vi "pidMotor.vi"(0 "Master refnum":string="My Motor RefNum", 5 "Slave refnum":string="My Motor RefNum", 7 "Joystick cluster":cluster{"X":dbl, "Y":dbl}, 9 "Speed Multiplier":dbl, 11 "error in (no error)":errorcluster) -> (4 "Set Velocity":dbl, 8 "Encoder Velocity":dbl, 15 "error out":errorcluster)   [LabVIEW 2014]
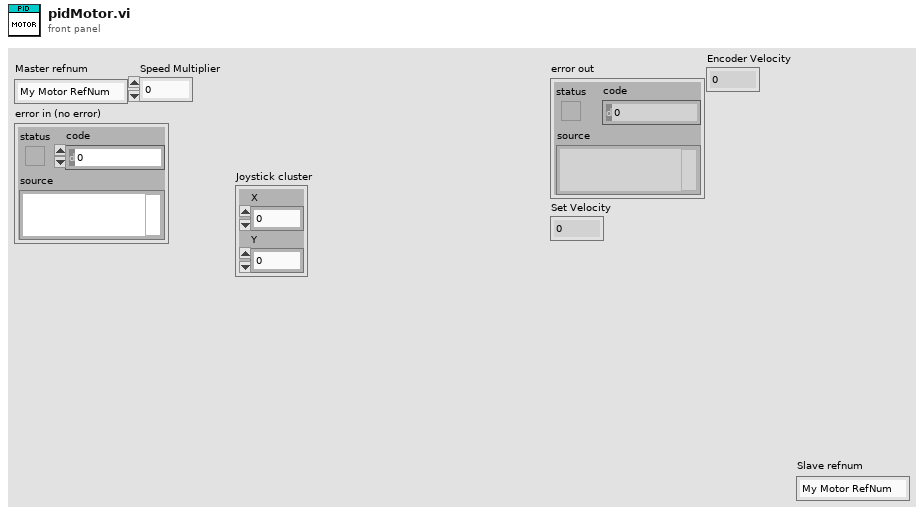
[diagram p1: front panel]
types:
  T1 = typedef "WPI_MotorControlDeviceRef.ctl" = cluster{"DeviceStatus":errorcluster, "Type":T2, "PWM":cluster{"Controller":T3, "PWM Channel":T4, "DeadBand":T5}, "CAN":cluster{"Device Number":u8, "Control Mode":T6, "Semaphore":T7, "Max Vout":dbl, "TalonSRX Control Mode":T8}, "Invert":bool, "TransformRef":T9, "InvTransformRef":T9}
  T2 = typedef "WPI_MotorControlType.ctl" = enum16{"PWM", "CAN", "CANTalonSRX"}
  T3 = typedef "FPGA_TypedefDigitalModule.ctl" = enum16{"Controller 1"}
  T4 = typedef "FPGA_DIOPWMChannel.ctl" = enum8{"PWM 0", "PWM 1", "PWM 2", "PWM 3", "PWM 4", "PWM 5", "PWM 6", "PWM 7", "PWM 8", "PWM 9", "PWM MXP 0", "PWM MXP 1", "PWM MXP 2", "PWM MXP 3", "PWM MXP 4", "PWM MXP 5", "PWM MXP 6", "PWM MXP 7", "PWM MXP 8", "PWM MXP 9", "Invalid"}
  T5 = typedef "WPI_PWMDeadband.ctl" = cluster{"Name":string, "maxPositivePwm":i32, "minPositivePwm":i32, "centerPwm":i32, "maxNegativePwm":i32, "minNegativePwm":i32, "angularRange":u16}
  T6 = typedef "WPI_CANJaguar_ControlMode.ctl" = enum8{"Percent VBus", "Current", "Speed", "Position", "Voltage"}
  T7 = typedef "Semaphore RefNum" = refnum<k1>
  T8 = typedef "WPI_CANTalonSRX_APIControlMode.ctl" = enum8{"Percent VBus", "Speed", "Position", "Slave", "Unchanged / Invalid"}
  T9 = typedef "WPI_PWMTransform_ConPane.ctl" = refnum<vi>
  T10 = typedef "WPI_CANTalonSRX_GlobalStatus.ctl" = cluster{"Applied Throttle":dbl, "Module Enabled":bool, "CAN Error":errorcluster, "Closed Loop Error":dbl, "Forward Limit Switch Closed":bool, "Reverse Limit Switch Closed":bool, "Sensor Position":dbl, "Sensor Velocity":dbl, "Current":dbl, "Sticky Fault - Over Temp":bool, "Sticky Fault - Under Voltage":bool, "Sticky Fault - Forward Limit":bool, "Sticky Fault - Reverse Limit":bool, "Sticky Fault - Forward Soft Limit":bool, "Sticky Fault - Reverse Soft Limit":bool, "Brake is Enabled":bool, "Encoder Position":dbl, "Encoder Velocity":dbl, "Encoder Index Count":dbl, "Encoder A Pin State":bool, "Encoder B Pin State":bool, "Encoder Index Pin State":bool, "Analog In":dbl, "Analog In Velocity":dbl, "Temperature (C)":dbl, "Battery Voltage":dbl}
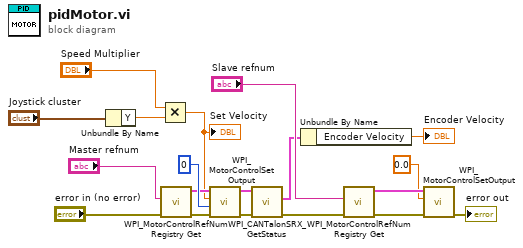
[diagram p0: block diagram]
diagram:
  n1 = Unbundle By Name("Joystick cluster") -> ("Y"=w5:dbl)
  n2 = Multiply(x="Speed Multiplier", y=w5) -> (x*y=w4:dbl)
  "Set Velocity" <- w4
  n3 = call <vilib>:"WPI_MotorControlRefNum Registry Get.vi"("error in (no error)"="error in (no error)", "refnum name"="Master refnum") -> ("error out"=w15:errorcluster, "MotorControlDevRef"=w13:T1)  [unwired: 8 in]
  n4 = call <vilib>:"WPI_MotorControlSetOutput.vi"("error in (no error)"=w15, "Sync Group / Parameter Slot"=u8 0, "Output"=w4, "MotorControlDevRef"=w13) -> ("error out"=w17:errorcluster, "MotorControlDevRef"=w16:T1)  [unwired: 5 in, 1 out]
  n5 = call <vilib>:"WPI_CANTalonSRX_GetStatus.vi"("error in (no error)"=w17, "CAN Talon SRX Ref"=w16) -> ("error out"=w7:errorcluster, "Talon SRX Status"=w2:T10)  [unwired: 7 in, 1 out]
  n6 = Unbundle By Name(w2) -> ("Encoder Velocity"=→"Encoder Velocity":dbl)
  n7 = call <vilib>:"WPI_MotorControlRefNum Registry Get.vi"("error in (no error)"=w7, "refnum name"="Slave refnum") -> ("error out"=w11:errorcluster, "MotorControlDevRef"=w10:T1)  [unwired: 8 in]
  n8 = call <vilib>:"WPI_MotorControlSetOutput.vi"("error in (no error)"=w11, "Output"=0.0, "MotorControlDevRef"=w10) -> ("error out"=→"error out":errorcluster)  [unwired: 6 in, 2 out]
